vi "fetchFromTarget.vi"(8 "error in (no error)":errorcluster, 10 "ConnectionData":T1, 11 "ConfigXMLControls":T2) -> (0 "error out":errorcluster, 1 "nameMessageOut":string, 2 "SuccessfulRead?":bool, 3 "path out":path)   [LabVIEW 2015]
uses:
  ConfigXMLControl.ctl
  General/RemoteFiles/connectionData.ctl
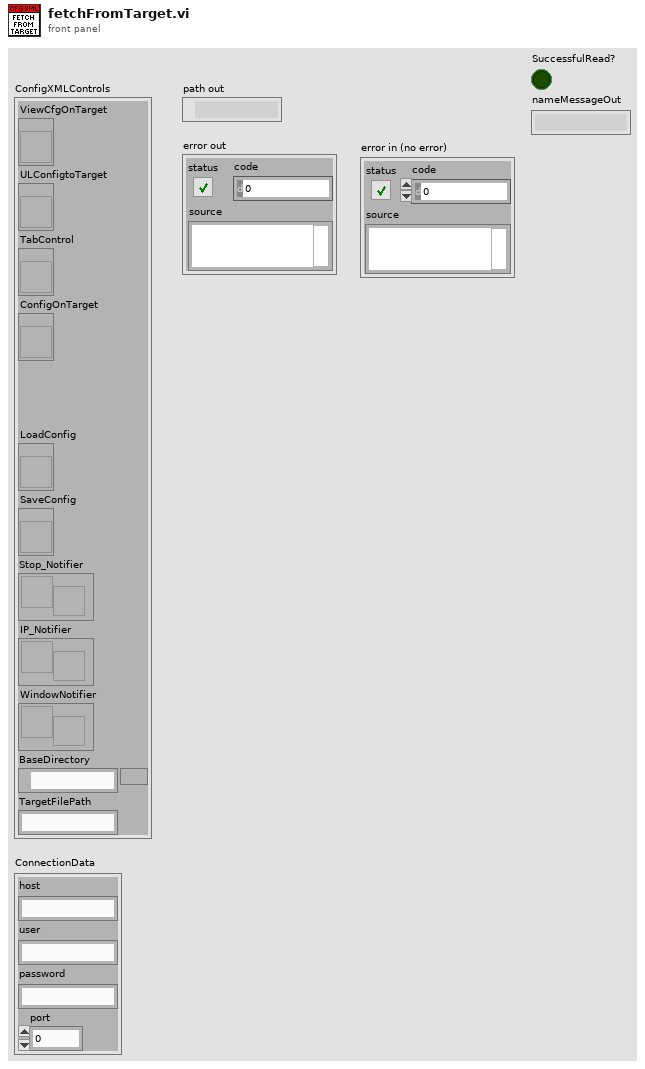
[diagram p1: front panel]
types:
  T1 = typedef "connectionData.ctl" = cluster{"host":string, "user":string, "password":string, "port":u16}
  T2 = typedef "ConfigXMLControl.ctl" = cluster{"ViewCfgOnTarget":refnum<vi>, "ULConfigtoTarget":refnum<vi>, "TabControl":refnum<vi>, "ConfigOnTarget":refnum<vi>, "LoadConfig":refnum<vi>, "SaveConfig":refnum<vi>, "Stop_Notifier":refnum<notifier>, "IP_Notifier":refnum<notifier>, "WindowNotifier":refnum<notifier>, "BaseDirectory":path, "TargetFilePath":string}
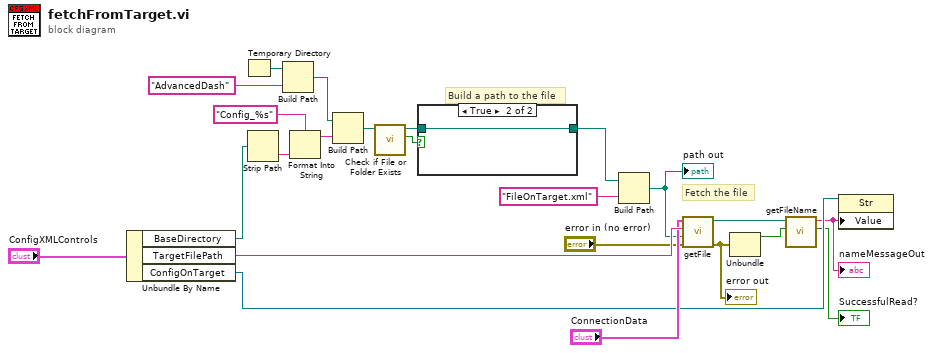
[diagram p0: block diagram]
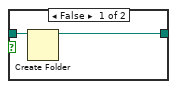
[diagram p2: hidden frame]
diagram:
  # "Build a path to the file"
  # "Fetch the file"
  n1 = Unbundle By Name("ConfigXMLControls") -> ("BaseDirectory"=w11:path, "TargetFilePath"=w23:string, "ConfigOnTarget"=w4:refnum<vi>)
  n2 = Temporary Directory() -> (w12:path)
  n3 = Strip Path(path=w11) -> (name=w17:string)  [unwired: 1 out]
  n4 = Build Path(base path=w12, name or relative path="AdvancedDash") -> (appended path=w14:path)
  n5 = Format Into String(format string="Config_%s", w17) -> (resulting string=w15:string)  [unwired: 2 in, 1 out]
  n6 = Build Path(base path=w14, name or relative path=w15) -> (appended path=w18:path)
  n7 = call <vilib>:"Check if File or Folder Exists.vi"("path"=w18) -> ("file or folder exists?"=w19:bool, "dup path"=w20:path)  [unwired: 8 in, 1 out]
  n8 = case shown="True" w19 {
    tunnel: w20 -> [w25 w26]
    tunnel: [w24 w26] -> w21
    frame False {
      n9 = Create Folder(path (use dialog)=w25) -> (created path=w24:path)  [unwired: 2 in, 2 out]
    }
    frame True {
    }
  }
  n10 = Build Path(base path=w21, name or relative path="FileOnTarget.xml") -> (appended path=w8:path)
  "path out" <- w8
  n11 = call "getFile.vi"("error in (no error)"="error in (no error)", "local path"=w8, "remote path"=w23, "ConnectionData"="ConnectionData") -> ("error out"=w5:errorcluster, "local path out"=w6:path)  [unwired: 6 in]
  "error out" <- w5
  n12 = Unbundle(w5) -> ("status"=w7:bool)  [unwired: 2 out]
  n13 = call "getFileName.vi"("File not found?"=w7, "Path"=w6) -> ("SuccessfulRead?"=→"SuccessfulRead?":bool, "Filename"=w3:string)  [unwired: 8 in]
  "nameMessageOut" <- w3
  n14 = property class="Str"(reference=w4, "Value"=w3) -> ()  [unwired: 1 in, 2 out]
